vi "BNO055 Read Reg.vi"(6 "Bytes To Read (1)":u8=1, 8 "error in (no error)":errorcluster, 9 "BNO055 Config Options":T1 {"ADC"."Comparator Queue & Disable" items=["Assert after one conversion", "Assert after two conversions", "Assert after four conversions", "Comparator disabled"]; "ADC"."Latching Comparator" items=["Non-latching", "Latching"]; "ADC"."Comparator Polarity" items=["Active Low", "Active High"]; "ADC"."Comparator Mode" items=["Traditional Comparator w/ hysteresis", "Window Comparator"]; "ADC"."Sampling Rate" items=["128SPS", "250SPS", "490SPS", "920SPS", "1600SPS", "2400SPS", "3300SPS"]; "ADC"."Sampling Mode" items=["Continuous Conversion", "Single-shot (Low Power)"]; "ADC"."Expected Range (Programmable Gain Amplifier)" items=["+/-6.144V", "+/-4.096V", "+/-2.048V", "+/-1.024V", "+/-0.512V", "+/-0.256V"]; "ADC"."Channel" items=["Differential: Ch 0&1", "Differential: Ch 0&3", "Differential: Ch 1&3", "Differential: Ch 2&3", "Single Ended: Ch 0", "Single Ended: Ch 1", "Single Ended: Ch 2", "Single Ended: Ch 3"]; "I2C"."Slave Address" format="%.0x"}, 10 "Register":u8 format="%.0x", 11 "LINX Resource in":T2) -> (0 "error out":errorcluster, 1 "BNO055 Config Options":T1 {"ADC"."Comparator Queue & Disable" items=["Assert after one conversion", "Assert after two conversions", "Assert after four conversions", "Comparator disabled"]; "ADC"."Latching Comparator" items=["Non-latching", "Latching"]; "ADC"."Comparator Polarity" items=["Active Low", "Active High"]; "ADC"."Comparator Mode" items=["Traditional Comparator w/ hysteresis", "Window Comparator"]; "ADC"."Sampling Rate" items=["128SPS", "250SPS", "490SPS", "920SPS", "1600SPS", "2400SPS", "3300SPS"]; "ADC"."Sampling Mode" items=["Continuous Conversion", "Single-shot (Low Power)"]; "ADC"."Expected Range (Programmable Gain Amplifier)" items=["+/-6.144V", "+/-4.096V", "+/-2.048V", "+/-1.024V", "+/-0.512V", "+/-0.256V"]; "ADC"."Channel" items=["Differential: Ch 0&1", "Differential: Ch 0&3", "Differential: Ch 1&3", "Differential: Ch 2&3", "Single Ended: Ch 0", "Single Ended: Ch 1", "Single Ended: Ch 2", "Single Ended: Ch 3"]; "I2C"."Slave Address" format="%.0x"}, 2 "Data out":u8[](array[numeric]), 3 "LINX Resource":T2)   [LabVIEW 2017]
uses:
  <vilib>/MakerHub/LINX/Private/Type Defs/Platform.ctl
  <vilib>/MakerHub/LINX/Private/Type Defs/Interface.ctl
  <vilib>/MakerHub/LINX/Private/Device/Type Defs/TCP Config.ctl
  <vilib>/MakerHub/LINX/Private/Device/Type Defs/Channels.ctl
  <vilib>/MakerHub/LINX/Private/Device/Type Defs/LINX Device Config.ctl
  <vilib>/MakerHub/LINX/Private/Type Defs/LINX Ref.ctl
  BNO055 Config Options.ctl
panel:
  # "NOT DONE\nYET!"
  # "NOT DONE\nYET!"
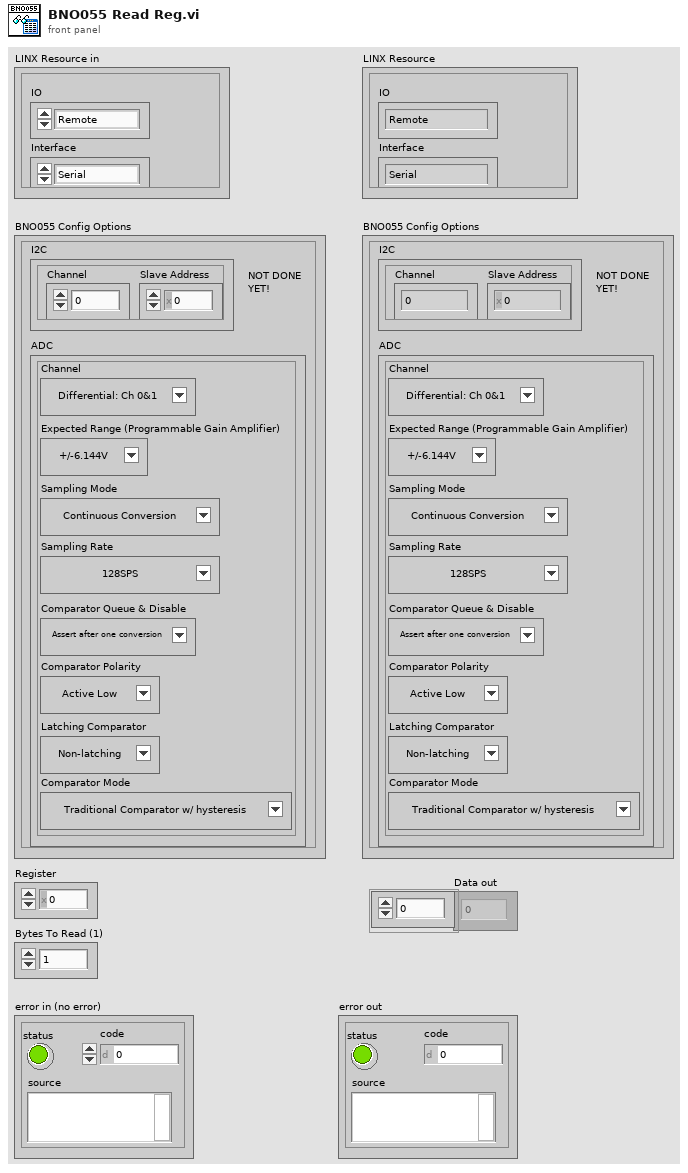
[diagram p1: front panel]
types:
  T1 = typedef "BNO055 Config Options.ctl" = cluster{"I2C":cluster{"Slave Address":u8, "Channel":u8}, "ADC":cluster{"Channel":u8, "Expected Range (Programmable Gain Amplifier)":u8, "Sampling Mode":u8, "Sampling Rate":u8, "Comparator Mode":u8, "Comparator Polarity":u8, "Latching Comparator":u8, "Comparator Queue & Disable":u8}}
  T2 = typedef "LMH-LINX.lvlib/LINX Ref.ctl" = cluster{"IO":T3, "Interface":T4, "LINX Device Config":T5}
  T3 = typedef "LMH-LINX.lvlib/Platform.ctl" = enum16{"Remote", "Local"}
  T4 = typedef "LMH-LINX.lvlib/Interface.ctl" = enum16{"Serial", "TCP"}
  T5 = typedef "LMH-LINX.lvlib/Device.lvlib/LINX Device Config.ctl" = cluster{"Interface":T4, "COM Port":refnum<visa-resource-name>, "TCP Configuration":T6, "Device Family":u8, "Device ID":u8, "Device Name":string, "TCP Ref":refnum<k5>, "Channels":T7}
  T6 = typedef "LMH-LINX.lvlib/Device.lvlib/TCP Config.ctl" = cluster{"IP Address":string, "Port":u16}
  T7 = typedef "LMH-LINX.lvlib/Channels.ctl" = cluster{"DI":u8[], "DO":u8[], "AI":u8[], "AO":u8[], "PWM":u8[], "QE":u8[], "UART":u8[], "I2C 2":u8[], "SPI":u8[], "CAN":u8[], "Servo":u8[], "AI Ref (V)":dbl, "AI Resolution (Bits)":u8, "AO Ref (V)":dbl, "AO Resolution (Bits)":u8}
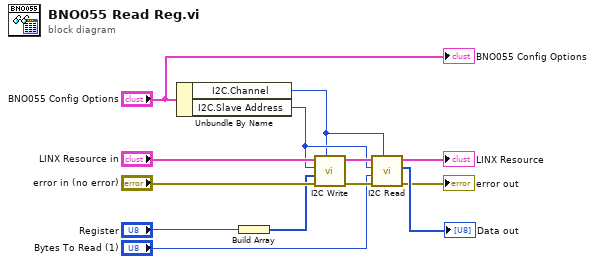
[diagram p0: block diagram]
diagram:
  n1 = Unbundle By Name("BNO055 Config Options") -> ("I2C.Channel"=w2:u8, "I2C.Slave Address"=w3:u8)
  n2 = Build Array("Register") -> (w4:u8[])
  n3 = call <vilib>:"I2C Write.vi"("I2C Channel"=w2, "Error In"="error in (no error)", "Data"=w4, "I2C Slave Address (0)"=w3, "LINX Resource"="LINX Resource in") -> ("Error Out"=w11:errorcluster, "LINX Resource"=w10:T2)  [unwired: 5 in]
  n4 = call <vilib>:"I2C Read.vi"("I2C Channel"=w2, "Error In"=w11, "Bytes To Read"="Bytes To Read (1)", "I2C Slave Address (0)"=w3, "LINX Resource"=w10) -> ("Error Out"=→"error out":errorcluster, "Data"=→"Data out":u8[], "LINX Resource"=→"LINX Resource":T2)  [unwired: 4 in]
  "BNO055 Config Options" <- "BNO055 Config Options"
